vi "Excel Get Data Specified Field.vi"(4 "error in (no error)":errorcluster, 5 "SheetName":string, 6 "file path":path, 7 "Start and End":T1) -> (0 "error out":errorcluster, 2 "data":string[][](array[string]), 3 "array":dbl[][](array[numeric]))   [LabVIEW 2011]
panel:
  in  "Excel._Worksheet 2":refnum<k7>
  in  "Array":string[][](array[string])
  in  "Excel._Worksheet":refnum<k7>
  in  "Excel._Application":refnum<k7>
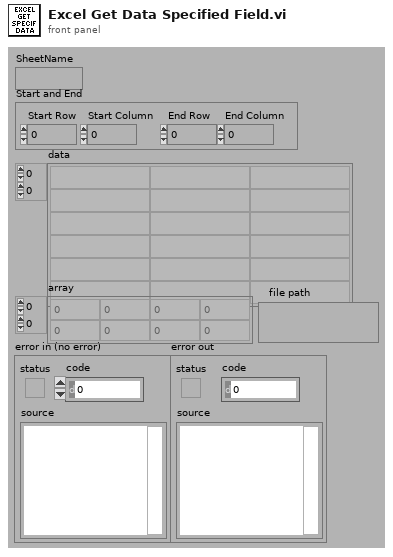
[diagram p1: front panel]
types:
  T1 = cluster{"Start Row":i32, "Start Column":i32, "End Row":i32, "End Column":i32}
  T2 = enum16{"open", "open or create", "create or replace", "create", "open (read only)"}
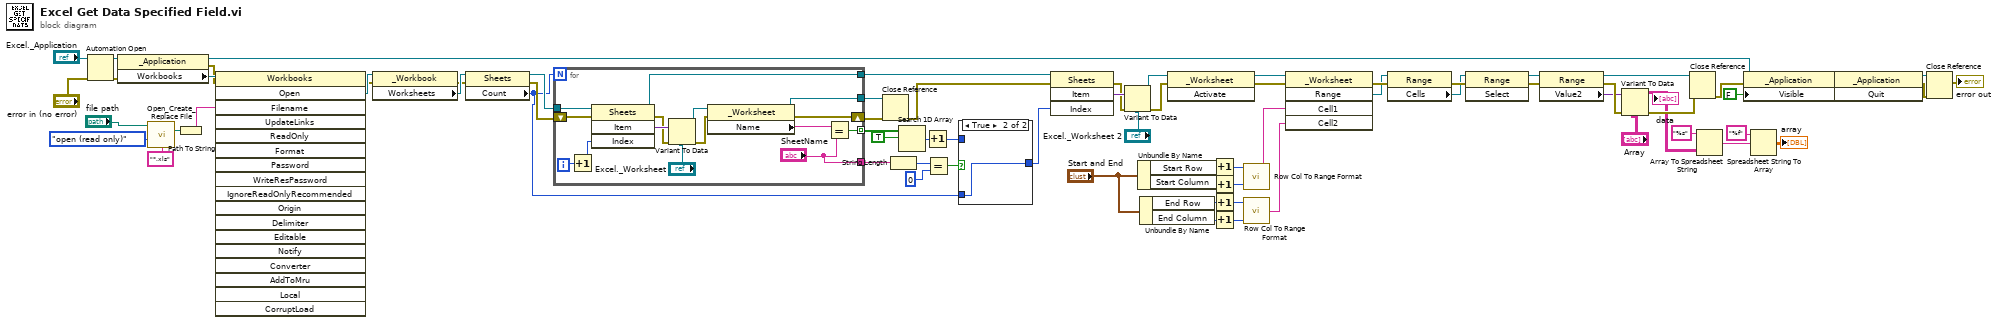
[diagram p0: block diagram]
diagram:
  n1 = Automation Open(error in (no error)="error in (no error)", Automation Refnum="Excel._Application") -> (Automation Refnum=w71:refnum<k7>, error out=w70:errorcluster)  [unwired: 2 out]
  n2 = property class="_Application"(reference=w71, error in=w70) -> (reference out=w61:refnum<k7>, error out=w64:errorcluster, "Workbooks"=w65:refnum<k7>)
  n3 = call <vilib>:"Open_Create_Replace File.vi"("pattern"="*.xls", "function (open:0)"=T2."open (read only)", "file path"="file path") -> ("new file path"=w28:path)  [unwired: 4 in, 4 out]
  n4 = Path To String(path=w28) -> (string=w9:string)
  n5 = invoke class="Workbooks" method="Open"(reference=w65, error in=w64, "Filename"=w9) -> (error out=w62:errorcluster, "Open"=w63:refnum<k7>)  [unwired: 15 in, 16 out]
  n6 = property class="_Workbook"(reference=w63, error in=w62) -> (error out=w49:errorcluster, "Worksheets"=w50:refnum<k7>)  [unwired: 1 out]
  n7 = property class="Sheets"(reference=w50, error in=w49) -> (reference out=w48:refnum<k7>, error out=w45:errorcluster, "Count"=w3:i32)
  n8 = for {
    N: w3 -> [_]
    tunnel: w48 -> [w88]
    shift-right: [w77] -> w41
    shift-left: w45 -> [w87]
    tunnel: [w78] -> w42 mode=indexing
    tunnel: [w76] -> w43
    tunnel: [w75] -> w39
    tunnel: ["SheetName"] -> w6
    i -> [w85]
    n9 = Increment(x=w85) -> (x+1=w86:i32)
    n10 = invoke class="Sheets" method="Item"(reference=w88, error in=w87, "Index"=w86) -> (reference out=w76:refnum<k7>, error out=w82:errorcluster, "Item"=w84:variant)  [unwired: 1 in, 1 out]
    n11 = Variant To Data(error in=w82, type="Excel._Worksheet", Variant=w84) -> (data=w80:refnum<k7>, error out=w81:errorcluster)
    n12 = property class="_Worksheet"(reference=w80, error in=w81) -> (reference out=w75:refnum<k7>, error out=w77:errorcluster, "Name"=w79:string)
    n13 = Equal?(x=w79, y="SheetName") -> (x = y?=w78:bool)
  }
  n14 = Close Reference(reference=w39, error in (no error)=w41) -> (error out=w40:errorcluster)
  n15 = String Length(string=w6) -> (length=w8:i32)
  n16 = Search 1D Array(1D array=w42, element=TRUE) -> (index of element=w46:i32)  [unwired: 1 out]
  n17 = Increment(x=w46) -> (x+1=w2:i32)
  n18 = Equal?(x=w8, y=0) -> (x = y?=w5:bool)
  n19 = case shown="True" w5 {
    tunnel: [w89 w90] -> w4
    tunnel: w3 -> [_ w90]
    tunnel: w2 -> [w89 _]
    frame False {
    }
    frame True {
    }
  }
  n20 = invoke class="Sheets" method="Item"(reference=w43, error in=w40, "Index"=w4) -> (error out=w68:errorcluster, "Item"=w69:variant)  [unwired: 1 in, 2 out]
  n21 = Variant To Data(error in=w68, type="Excel._Worksheet 2", Variant=w69) -> (data=w38:refnum<k7>, error out=w67:errorcluster)
  n22 = Unbundle By Name("Start and End") -> ("Start Row"=w21:i32, "Start Column"=w20:i32)
  n23 = Unbundle By Name("Start and End") -> ("End Row"=w19:i32, "End Column"=w18:i32)
  n24 = invoke class="_Worksheet" method="Activate"(reference=w38, error in=w67) -> (reference out=w26:refnum<k7>, error out=w25:errorcluster)  [unwired: 1 in, 1 out]
  n25 = Increment(x=w21) -> (x+1=w23:i32)
  n26 = Increment(x=w20) -> (x+1=w24:i32)
  n27 = Increment(x=w19) -> (x+1=w17:i32)
  n28 = Increment(x=w18) -> (x+1=w16:i32)
  n29 = call "Row Col To Range Format.vi"("Column"=w24, "Row"=w23) -> ("Output String"=w15:string)
  n30 = call "Row Col To Range Format.vi"("Column"=w16, "Row"=w17) -> ("Output String"=w14:string)
  n31 = invoke class="_Worksheet" method="Range"(reference=w26, error in=w25, "Cell1"=w15, "Cell2"=w14) -> (error out=w13:errorcluster, "Range"=w12:refnum<k7>)  [unwired: 1 in, 3 out]
  n32 = property class="Range"(reference=w12, error in=w13) -> (error out=w58:errorcluster, "Cells"=w37:refnum<k7>)  [unwired: 1 out]
  n33 = invoke class="Range" method="Select"(reference=w37, error in=w58) -> (reference out=w57:refnum<k7>, error out=w56:errorcluster)  [unwired: 1 in, 1 out]
  n34 = property class="Range"(reference=w57, error in=w56) -> (reference out=w54:refnum<k7>, error out=w55:errorcluster, "Value2"=w51:variant)
  n35 = Variant To Data(error in=w55, type="Array", Variant=w51) -> (data=w11:string[][], error out=w53:errorcluster)
  "data" <- w11
  n36 = Close Reference(reference=w54, error in (no error)=w53) -> (error out=w52:errorcluster)
  n37 = Array To Spreadsheet String(array=w11, 3:"%s" ("format string")) -> (spreadsheet string=w32:string)  [unwired: 1 out]
  n38 = property class="_Application"(reference=w61, error in=w52, "Visible"=FALSE) -> (reference out=w59:refnum<k7>, error out=w60:errorcluster)
  n39 = Spreadsheet String To Array(format string="%f", spreadsheet string=w32) -> (array=→"array":dbl[][])  [unwired: 2 out]
  n40 = invoke class="_Application" method="Quit"(reference=w59, error in=w60) -> (reference out=w36:refnum<k7>, error out=w35:errorcluster)  [unwired: 1 in, 1 out]
  n41 = Close Reference(reference=w36, error in (no error)=w35) -> (error out=→"error out":errorcluster)
